vi "From String Array.vi"(0 "Data":cluster{"Key":string, "Value":string}[](array[cluster])) -> (2 "Map":refnum<class "Map.lvclass">)   [LabVIEW 2018, in "Toolkit.lvlib" / "Data.lvlib" / "Map.lvclass"]
uses:
  Map.lvclass
  Map.lvclass/Map.ctl
  String/String.lvclass
  D:/Users/cfield/Code/Field R&D Services/Mustache/trunk/src/Toolkit/Data/Abstract/Abstract.lvclass
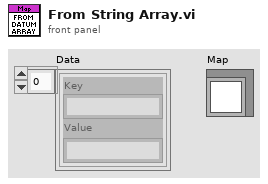
[diagram p1: front panel]
types:
  T1 = cluster{"Key":string, "String":refnum<class "String.lvclass">}
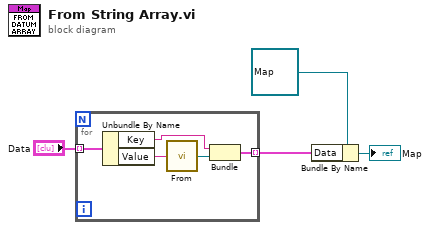
[diagram p0: block diagram]
diagram:
  n1 = for {
    tunnel: "Data" -> [w9] mode=indexing
    tunnel: [w5] -> w1 mode=indexing
    n2 = Unbundle By Name(w9) -> ("Key"=w7:string, "Value"=w8:string)
    n3 = call "From.vi"("Value"=w8) -> ("String"=w6:refnum<class "String.lvclass">)
    n4 = Bundle("Key"=w7, "String"=w6) -> (w5:T1)  [unwired: 1 in]
  }
  n5 = Bundle By Name(cluster=refnum<class "Map.lvclass"> refnum ("Toolkit.lvlib:Data.lvlib:Map.lvclass"), "Data"=w1) -> (→"Map":refnum<class "Map.lvclass">)
